vi "Main.vi"() -> ()   [LabVIEW 2014]
doc: "Program główny. (Jak narazie)\nTime w kliencie można interpretować jako sekundy (nie jest to oczywiste, bo ma typ double)."
uses:
  Client.ctl
  Kasy.ctl
  LukiBrary.lvlib
panel:
  out "Waveform Chart":i32(graph)
  out "# elements in queue":i32
  out "Obsługiwanych klientów":i32
  out "Kasa 2":T1
  in  "Max czas obsługi":dbl
  in  "Kasa":T1={"Zarobek"=0.0, "Liczba kas"=4, "Czas"=[]}
  out "People":T2[](array[typedef])
  in  "lambda":dbl=1.0 format="%#_13g"
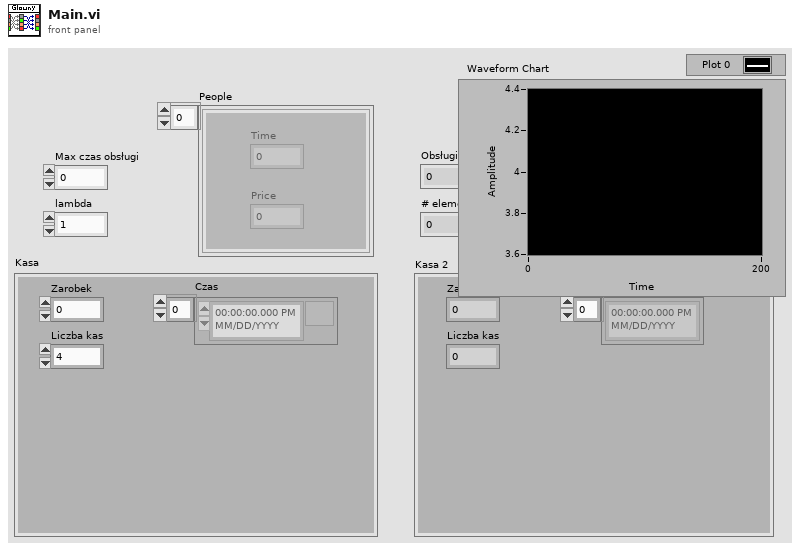
[diagram p1: front panel]
types:
  T1 = typedef "Kasy.ctl" = cluster{"Zarobek":dbl, "Liczba kas":u8, "Czas":timestamp[]}
  T2 = typedef "LukiBrary.lvlib/Client.ctl" = cluster{"Time":dbl, "Price":dbl}
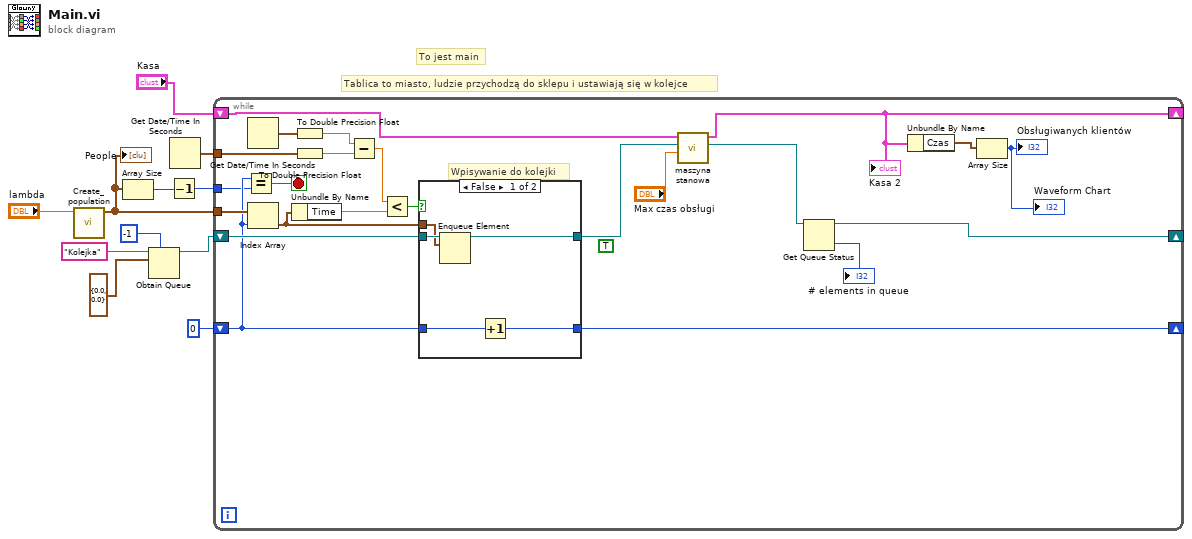
[diagram p0: block diagram]
diagram:
  # "To jest main"
  # "Tablica to miasto, ludzie przychodzą do sklepu i ustawiają się w kolejce"
  n1 = call "Create_population.vi"("lambda"="lambda") -> ("People"=w4:T2[])  [unwired: 10 in]
  "People" <- w4
  n2 = Array Size(array=w4) -> (size(s)=w3:i32)
  n3 = Obtain Queue(max queue size (-1, unlimited)=-1, name (unnamed)="Kolejka", element data type=T2 {"Time"=0.0, "Price"=0.0} ("Client")) -> (queue out=w5:refnum<queue>)  [unwired: 2 in, 2 out]
  n4 = Decrement(x=w3) -> (x-1=w2:i32)
  n5 = Get Date/Time In Seconds() -> (seconds since 1Jan1904=w9:timestamp)
  n6 = while {
    tunnel: w4 -> [w34]
    shift-right: [w25] -> _
    shift-left: 0 -> [w23]
    tunnel: w9 -> [w33]
    shift-right: [w14] -> _
    shift-left: w5 -> [w24]
    tunnel: w2 -> [w22]
    shift-right: [w16] -> _
    shift-left: "Kasa" -> [w20]
    stop <- w21 stop-if-true
    (unwired) TRUE ("return elements? (F)")
    # "Wpisywanie do kolejki"
    n7 = Equal?(x=w23, y=w22) -> (x = y?=w21:bool)
    n8 = Get Date/Time In Seconds() -> (seconds since 1Jan1904=w32:timestamp)
    n9 = Index Array(array=w34, index=w23) -> (element=w26:T2)
    n10 = Unbundle By Name(w26) -> ("Time"=w29:dbl)
    n11 = To Double Precision Float(number=w32) -> (double precision float=w31:dbl)
    n12 = To Double Precision Float(number=w33) -> (double precision float=w30:dbl)
    n13 = Subtract(x=w31, y=w30) -> (x-y=w28:dbl)
    n14 = Less?(x=w28, y=w29) -> (x < y?=w27:bool)
    n15 = case shown="False" w27 {
      tunnel: w23 -> [w39 w41]
      tunnel: [w38 w41] -> w25
      tunnel: w26 -> [w35 _]
      tunnel: w24 -> [w37 w40]
      tunnel: [w36 w40] -> w18
      frame False {
        n16 = Enqueue Element(queue=w37, element=w35) -> (queue out=w36:refnum<queue>)  [unwired: 2 in, 2 out]
        n17 = Increment(x=w39) -> (x+1=w38:i32)
      }
      frame True {
      }
    }
    n18 = call "maszyna stanowa.vi"("Max czas obsługi"="Max czas obsługi", "Queue in"=w18, "Kasa"=w20) -> ("Queue in 2"=w17:refnum<queue>, "Kasa 2"=w16:T1)  [unwired: 7 in]
    "Kasa 2" <- w16
    n19 = Get Queue Status(queue=w17) -> (queue out=w14:refnum<queue>, # elements in queue=→"# elements in queue":i32)  [unwired: 2 in, 6 out]
    n20 = Unbundle By Name(w16) -> ("Czas"=w15:timestamp[])
    n21 = Array Size(array=w15) -> (size(s)=→"Obsługiwanych klientów" →"Waveform Chart":i32)
  }
